vi "Insert Coin.vi"(0 "reference in":refnum<class "Sold State.lvclass">, 5 "error in (no error)":errorcluster) -> (14 "reference out":refnum<class "Sold State.lvclass">, 19 "error out":errorcluster)   [LabVIEW 2013, in "Sold State.lvclass"]
uses:
  Sold State.lvclass
  Gum Machine_class/Gum Machine.lvclass
panel:
  out "Gum Machine.lvclass":refnum<class "Gum Machine.lvclass">
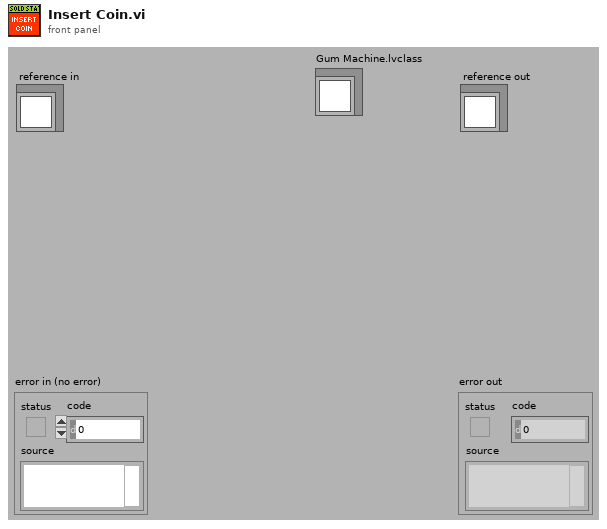
[diagram p1: front panel]
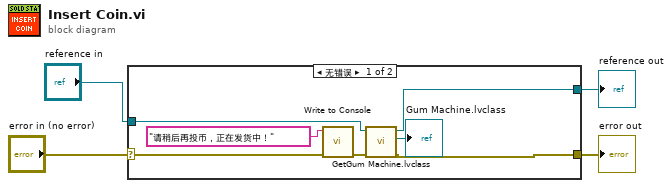
[diagram p0: block diagram]
diagram:
  n1 = case shown="无错误" "error in (no error)" {
    selector: "error in (no error)" -> [w8 w13]
    tunnel: [w6 w13] -> w3
    tunnel: [w9 w12] -> w1
    tunnel: "reference in" -> [w10 w12]
    frame No Error {
      n2 = call "Write to Console.vi"("error in (no error)"=w8, "Input"="请稍后再投币，正在发货中！") -> ("error out"=w7:errorcluster)  [unwired: 9 in]
      n3 = call-dynamic "GetGum Machine.lvclass.vi"("error in (no error)"=w7, "reference in"=w10) -> ("error out"=w6:errorcluster, "Gum Machine.lvclass"=→"Gum Machine.lvclass":refnum<class "Gum Machine.lvclass">, "reference out"=w9:refnum<class "Sold State.lvclass">)  [unwired: 7 in]
    }
    frame Error {
    }
  }
  "error out" <- w3
  "reference out" <- w1
